vi "CAN Read Timeout.vi"(8 "error in (no error)":errorcluster, 9 "Timeout (ms)":u32, 10 "Message ID Mask":u32=4294967295 format="%.0x", 11 "Message ID":u32 format="%.0x") -> (0 "error out":errorcluster, 3 "data":u8[](array[numeric]), 4 "timestamp":u32)   [LabVIEW 2023]
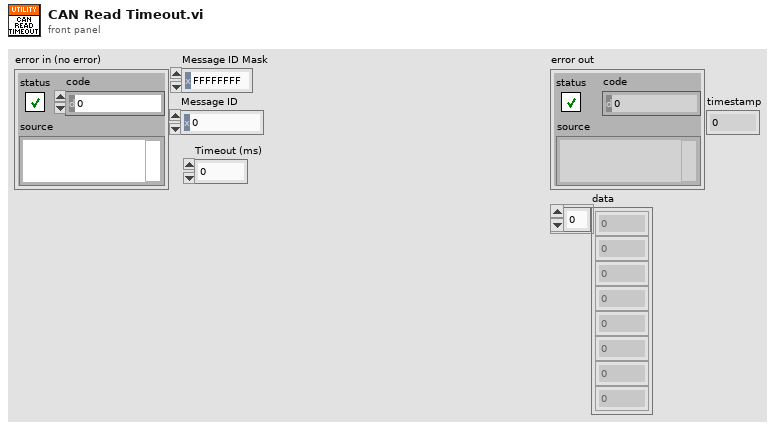
[diagram p1: front panel]
types:
  T1 = map{u32, cluster{"timestamp":u32, "data":u8[], "length":u8}}
  T2 = cluster{"timestamp":u32, "data":u8[], "length":u8}
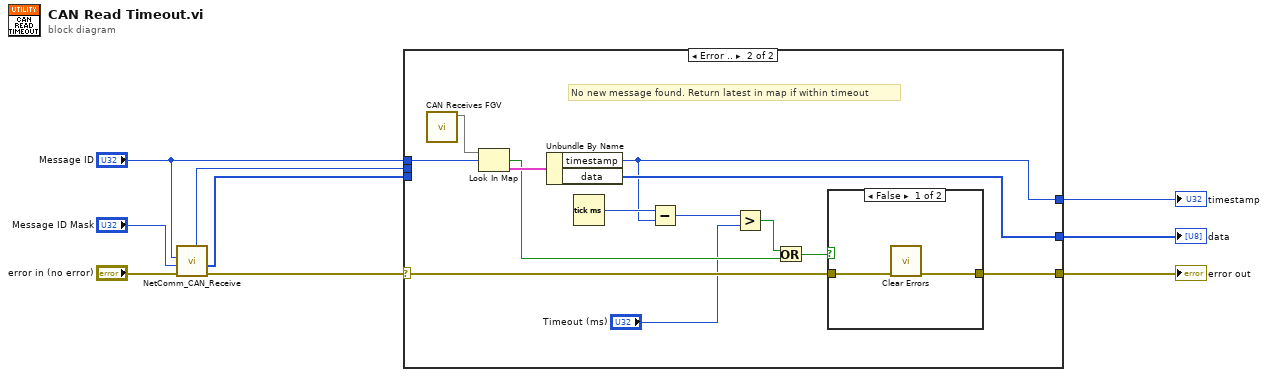
[diagram p0: block diagram]
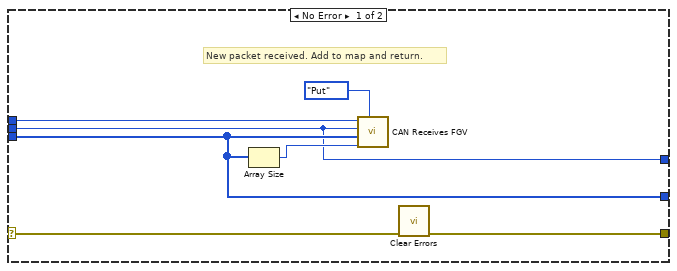
[diagram p2: hidden frame]
diagram:
  n1 = call <vilib>:"NetComm_CAN_Receive.vi"("error in (no error)"="error in (no error)", "Message ID Mask"="Message ID Mask", "Message ID"="Message ID") -> ("error out"=w7:errorcluster, "Data"=w4:u8[], "timeStamp"=w5:u32)  [unwired: 6 out]
  n2 = case shown="Error .." w7 {
    selector: w7 -> [w12 w25]
    tunnel: "Message ID" -> [w16 w28]
    tunnel: w5 -> [w10 _]
    tunnel: w4 -> [w13 _]
    tunnel: [w13 w26] -> w3
    tunnel: [w11 w24] -> w2
    tunnel: [w10 w21] -> w1
    frame No Error {
      # "New packet received. Add to map and return."
      n3 = Array Size(array=w13) -> (size(s)=w14:i32)
      n4 = call "CAN Receives FGV.vi"("Action"=enum16{"Get", "Put"}."Put", "length"=w14, "data"=w13, "timestamp"=w10, "arb id"=w16) -> ()  [unwired: 6 in, 1 out]
      n5 = call <vilib>:"Clear Errors.vi"("error in (no error)"=w12) -> ("error out"=w11:errorcluster)  [unwired: 5 in, 1 out]
    }
    frame Error {
      # "No new message found. Return latest in map if within timeout"
      n6 = call "CAN Receives FGV.vi"() -> ("Receives"=w29:T1)  [unwired: 11 in]
      n7 = Look In Map(map=w29, key=w28) -> (key not found?=w23:bool, value=w27:T2)  [unwired: 1 in]
      n8 = Unbundle By Name(w27) -> ("timestamp"=w21:u32, "data"=w26:u8[])
      n9 = Tick Count (ms)() -> (millisecond timer value=w22:u32)
      n10 = Subtract(x=w22, y=w21) -> (x-y=w20:u32)
      n11 = Greater?(x=w20, y="Timeout (ms)") -> (0:w18:bool)
      n12 = Or(x=w18, y=w23) -> (x .or. y?=w17:bool)
      n13 = case shown="False" w17 {
        tunnel: w25 -> [w31 w32]
        tunnel: [w30 w32] -> w24
        frame False {
          n14 = call <vilib>:"Clear Errors.vi"("error in (no error)"=w31) -> ("error out"=w30:errorcluster)  [unwired: 5 in, 1 out]
        }
        frame True {
        }
      }
    }
  }
  "error out" <- w2
  "data" <- w3
  "timestamp" <- w1
